vi "索引数组.vi"() -> ()   [LabVIEW 2018]
panel:
  out "元素":dbl
  in  "索引号":dbl
  in  "数组":dbl[](array[numeric])
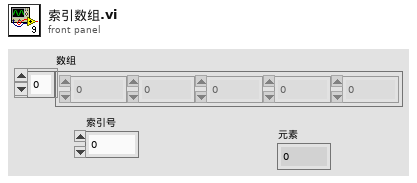
[diagram p1: front panel]
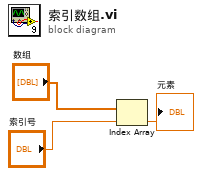
[diagram p0: block diagram]
diagram:
  n1 = Index Array(array="数组", index="索引号") -> (element=→"元素":dbl)
